vi "Stop or Full Quit if compiled.vi"(1 "error in (no effect)":errorcluster, 2 "stop/quit? (T)":bool=TRUE) -> ()   [LabVIEW 2020, in "varilib.lvlib"]
doc: "If <b>not</b> in Run Time System: Stops the VI in which it executes, just as if you clicked the Abort Execution button on the toolbar. (Does not close all VIs, does not close LabVIEW).\nIf <b>in</b> Run Time System (compiled executable): Stops all executing VIs and ends the current instance of LabVIEW. (Close all VIs, stops the exe program).\nError in has no effect, it is only for synchronization of blocks execution."
uses:
  varilib.lvlib
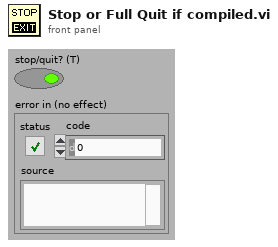
[diagram p1: front panel]
types:
  T1 = enum32{"invalid app kind", "Development System", "Run Time System", "Student Edition", "Embedded LabVIEW", "Evaluation", "Custom"}
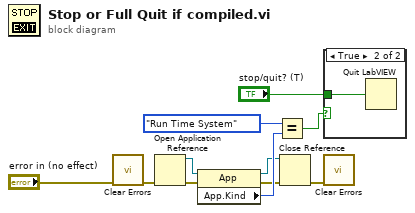
[diagram p0: block diagram]
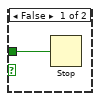
[diagram p2: hidden frame]
diagram:
  n1 = call <vilib>:"Clear Errors.vi"("error in (no error)"="error in (no effect)") -> ("error out"=w1:errorcluster)  [unwired: 5 in, 1 out]
  n2 = Open Application Reference(8:w1) -> (0:w8:errorcluster, 3:w11:refnum<vi>)  [unwired: 3 in]
  n3 = property class="App"(reference=w11, error in=w8) -> (reference out=w6:refnum<vi>, error out=w7:errorcluster, "App.Kind"=w9:T1)
  n4 = Equal?(x=T1."Run Time System" ("Application:Kind"), y=w9) -> (x = y?=w4:bool)
  n5 = Close Reference(reference=w6, error in (no error)=w7) -> (error out=w5:errorcluster)
  n6 = case shown="True" w4 {
    tunnel: "stop/quit? (T)" -> [w12 w13]
    frame False {
      n7 = Stop(stop? (T)=w12) -> ()
    }
    frame True {
      n8 = Quit LabVIEW(quit? (T)=w13) -> ()
    }
  }
  n9 = call <vilib>:"Clear Errors.vi"("error in (no error)"=w5) -> ()  [unwired: 5 in, 2 out]
